vi "Debug_Convert_Data_to_String.vi"(8 "error in (no error)":errorcluster, 11 "AB_InteropAssembly in":refnum<class "AB_InteropAssembly.lvclass">) -> (0 "error out":errorcluster, 2 "classData":string, 3 "AB_InteropAssembly out":refnum<class "AB_InteropAssembly.lvclass">)   [LabVIEW 2020, in "AB_InteropAssembly.lvclass"]
uses:
  <vilib>/AppBuilder/AB_Classes/InteropAssembly/AB_InteropAssembly.lvclass
  <vilib>/AppBuilder/AB_Classes/InteropAssembly/AB_InteropAssembly.lvclass/AB_InteropAssembly.ctl
  <vilib>/AppBuilder/AB_Classes/Application/AB_Application.lvclass
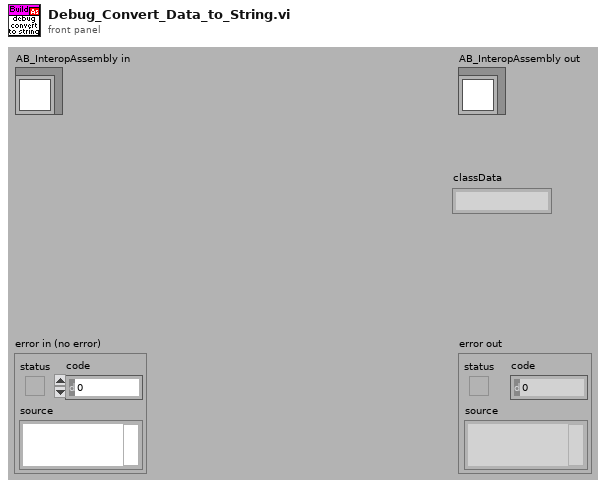
[diagram p1: front panel]
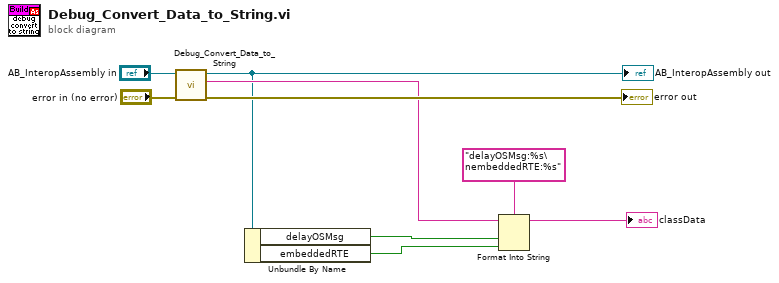
[diagram p0: block diagram]
diagram:
  n1 = call-parent "Debug_Convert_Data_to_String.vi"("error in (no error)"="error in (no error)", "AB_Application in"="AB_InteropAssembly in") -> ("error out"=→"error out":errorcluster, "classData"=w6:string, "AB_Application out"=w1:refnum<class "AB_InteropAssembly.lvclass">)  [unwired: 7 out]
  "AB_InteropAssembly out" <- w1
  n2 = Unbundle By Name(w1) -> ("delayOSMsg"=w4:bool, "embeddedRTE"=w3:bool)
  n3 = Format Into String(format string="delayOSMsg:%s\nembeddedRTE:%s", initial string=w6, w4, w3) -> (resulting string=→"classData":string)  [unwired: 1 in, 1 out]
